vi "readFoodInfo.vi"() -> (0 "数组":cluster{"ID":dbl, "食品名称":string, "价格":dbl}[](array[cluster]))   [LabVIEW 2013, in "FoodBase.lvclass"]
uses:
  FoodBase.lvclass
  <vilib>/Utility/xml.llb/Read From XML File(string).vi
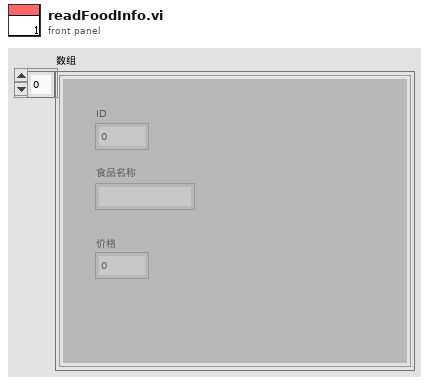
[diagram p1: front panel]
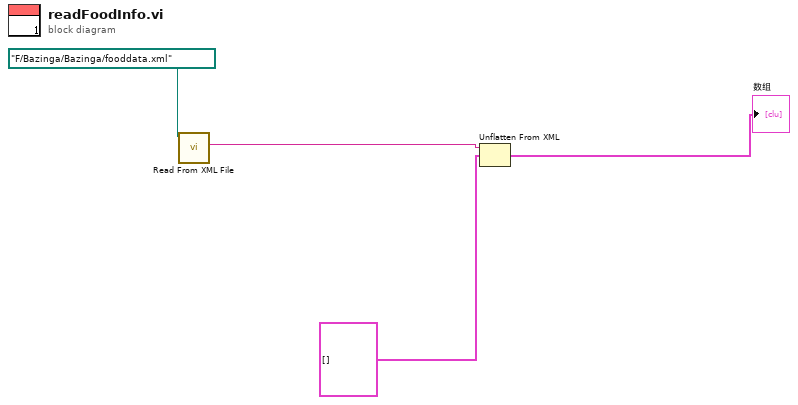
[diagram p0: block diagram]
diagram:
  n1 = call-poly <vilib>:"Read From XML File.vi"("XML File Path"=path "F:/Bazinga/Bazinga/fooddata.xml") -> ("XML Elements"=w2:string)  [unwired: 8 in, 2 out]
  n2 = Unflatten From XML(xml string=w2, type=cluster{"ID":dbl, "食品名称":string, "价格":dbl}[] [] ("数组 2")) -> (value=→"数组":cluster{"ID":dbl, "食品名称":string, "价格":dbl}[])  [unwired: 1 in, 1 out]
